vi "Format Commands to Tree.vi"(8 "Paths":path[](array[path])=[path "C:/Users/gam.AMER/Documents/2468 code/trunk/FRC/2019/Software/2019 robot/Drive/Commands/Drive for Time.vi", path "C:/Users/gam.AMER/Documents/2468 code/trunk/FRC/2019/Software/2019 robot/Drive/Commands/Drive Immediate.vi", path "C:/Users/gam.AMER/Documents/2468 code/trunk/FRC/2019/Software/2019 robot/Drive/Commands/J-Turn.vi", path "C:/Users/gam.AMER/Documents/2468 code/trunk/FRC/2019/Software/2019 robot/Drive/Commands/Play Path.vi", path "C:/Users/gam.AMER/Documents/2468 code/trunk/FRC/2019/Software/2019 robot/Drive/Commands/Read Drive Operation.vi", path "C:/Users/gam.AMER/Documents/2468 code/trunk/FRC/2019/Software/2019 robot/Drive/Commands/Reserve Drive.vi", path "C:/Users/gam.AMER/Documents/2468 code/trunk/FRC/2019/Software/2019 robot/Drive/Commands/Stop Driving.vi", path "C:/Users/gam.AMER/Documents/2468 code/trunk/FRC/2019/Software/2019 robot/Drive/Commands/Template for Drive Immediate with Deadband.vit", path "C:/Users/gam.AMER/Documents/2468 code/trunk/FRC/2019/Software/2019 robot/Drive/Commands/Template for Drive Immediate.vit", path "C:/Users/gam.AMER/Documents/2468 code/trunk/FRC/2019/Software/2019 robot/Drive/Commands/Template for Drive with Duration.vit", path "C:/Users/gam.AMER/Documents/2468 code/trunk/FRC/2019/Software/2019 robot/Climb/Commands/climb.vi", path "C:/Users/gam.AMER/Documents/2468 code/trunk/FRC/2019/Software/2019 robot/Climb/Commands/Read Climb Operation.vi", path "C:/Users/gam.AMER/Documents/2468 code/trunk/FRC/2019/Software/2019 robot/Climb/Commands/Reserve Climb.vi", path "C:/Users/gam.AMER/Documents/2468 code/trunk/FRC/2019/Software/2019 robot/Climb/Commands/Template for Climb Immediate with Deadband.vit", path "C:/Users/gam.AMER/Documents/2468 code/trunk/FRC/2019/Software/2019 robot/Climb/Commands/Template for Climb Immediate.vit", path "C:/Users/gam.AMER/Documents/2468 code/trunk/FRC/2019/Software/2019 robot/Climb/Commands/Template for Climb with Duration.vit", path "C:/Users/gam.AMER/Documents/2468 code/trunk/FRC/2019/Software/2019 robot/Elevator/Commands/Elevator Immediate.vi", path "C:/Users/gam.AMER/Documents/2468 code/trunk/FRC/2019/Software/2019 robot/Elevator/Commands/Read Elevator Operation.vi", path "C:/Users/gam.AMER/Documents/2468 code/trunk/FRC/2019/Software/2019 robot/Elevator/Commands/Reserve Elevator.vi", path "C:/Users/gam.AMER/Documents/2468 code/trunk/FRC/2019/Software/2019 robot/Elevator/Commands/Template for Elevator Immediate with Deadband.vit", path "C:/Users/gam.AMER/Documents/2468 code/trunk/FRC/2019/Software/2019 robot/Elevator/Commands/Template for Elevator Immediate.vit", path "C:/Users/gam.AMER/Documents/2468 code/trunk/FRC/2019/Software/2019 robot/Elevator/Commands/Template for Elevator with Duration.vit", path "C:/Users/gam.AMER/Documents/2468 code/trunk/FRC/2019/Software/2019 robot/Floating Intake/Commands/Duration Intake.vi", path "C:/Users/gam.AMER/Documents/2468 code/trunk/FRC/2019/Software/2019 robot/Floating Intake/Commands/Floating Intake Immediate.vi", path "C:/Users/gam.AMER/Documents/2468 code/trunk/FRC/2019/Software/2019 robot/Floating Intake/Commands/Floating Intake Read.vi", path "C:/Users/gam.AMER/Documents/2468 code/trunk/FRC/2019/Software/2019 robot/Floating Intake/Commands/Read Floating Intake Operation.vi", path "C:/Users/gam.AMER/Documents/2468 code/trunk/FRC/2019/Software/2019 robot/Floating Intake/Commands/Reserve Floating Intake.vi", path "C:/Users/gam.AMER/Documents/2468 code/trunk/FRC/2019/Software/2019 robot/Floating Intake/Commands/Template for Floating Intake Immediate with Deadband.vit", path "C:/Users/gam.AMER/Documents/2468 code/trunk/FRC/2019/Software/2019 robot/Floating Intake/Commands/Template for Floating Intake Immediate.vit", path "C:/Users/gam.AMER/Documents/2468 code/trunk/FRC/2019/Software/2019 robot/Floating Intake/Commands/Template for Floating Intake with Duration.vit", path "C:/Users/gam.AMER/Documents/2468 code/trunk/FRC/2019/Software/2019 robot/Carriage Intake/Commands/Carriage Intake Immediate with Deadband.vi", path "C:/Users/gam.AMER/Documents/2468 code/trunk/FRC/2019/Software/2019 robot/Carriage Intake/Commands/Carriage Intake Immediate.vi", path "C:/Users/gam.AMER/Documents/2468 code/trunk/FRC/2019/Software/2019 robot/Carriage Intake/Commands/Read Carriage Intake Operation.vi", path "C:/Users/gam.AMER/Documents/2468 code/trunk/FRC/2019/Software/2019 robot/Carriage Intake/Commands/Reserve Carriage Intake.vi", path "C:/Users/gam.AMER/Documents/2468 code/trunk/FRC/2019/Software/2019 robot/Carriage Intake/Commands/Template for Carriage Intake Immediate with Deadband.vit", path "C:/Users/gam.AMER/Documents/2468 code/trunk/FRC/2019/Software/2019 robot/Carriage Intake/Commands/Template for Carriage Intake Immediate.vit", path "C:/Users/gam.AMER/Documents/2468 code/trunk/FRC/2019/Software/2019 robot/Carriage Intake/Commands/Template for Carriage Intake with Duration.vit", path "C:/Users/gam.AMER/Documents/2468 code/trunk/FRC/2019/Software/2019 robot/LattePanda/Commands/Is Connected.vi", path "C:/Users/gam.AMER/Documents/2468 code/trunk/FRC/2019/Software/2019 robot/LattePanda/Commands/Power On.vi", path "C:/Users/gam.AMER/Documents/2468 code/trunk/FRC/2019/Software/2019 robot/LattePanda/Commands/Read LattePanda Operation.vi", path "C:/Users/gam.AMER/Documents/2468 code/trunk/FRC/2019/Software/2019 robot/LattePanda/Commands/Reserve LattePanda.vi", path "C:/Users/gam.AMER/Documents/2468 code/trunk/FRC/2019/Software/2019 robot/LattePanda/Commands/Shut Down.vi", path "C:/Users/gam.AMER/Documents/2468 code/trunk/FRC/2019/Software/2019 robot/LattePanda/Commands/Template for LattePanda Immediate with Deadband.vit", path "C:/Users/gam.AMER/Documents/2468 code/trunk/FRC/2019/Software/2019 robot/LattePanda/Commands/Template for LattePanda Immediate.vit", path "C:/Users/gam.AMER/Documents/2468 code/trunk/FRC/2019/Software/2019 robot/LattePanda/Commands/Template for LattePanda with Duration.vit"], 9 "Command Info":T4(array[cluster]), 11 "Tree Refnum":refnum<vi>) -> (2 "2D Picture":picture, 3 "Filtered Command Info Out":T1)   [LabVIEW 2019]
uses:
  <vilib>/picture/picture.llb/imagedata.ctl
  Command Editor Info.ctl
  Single Cmd Info.ctl
  <vilib>/Utility/Data Type/NI_Data Type.lvlib
panel:
  in  "Tree":string(tree)
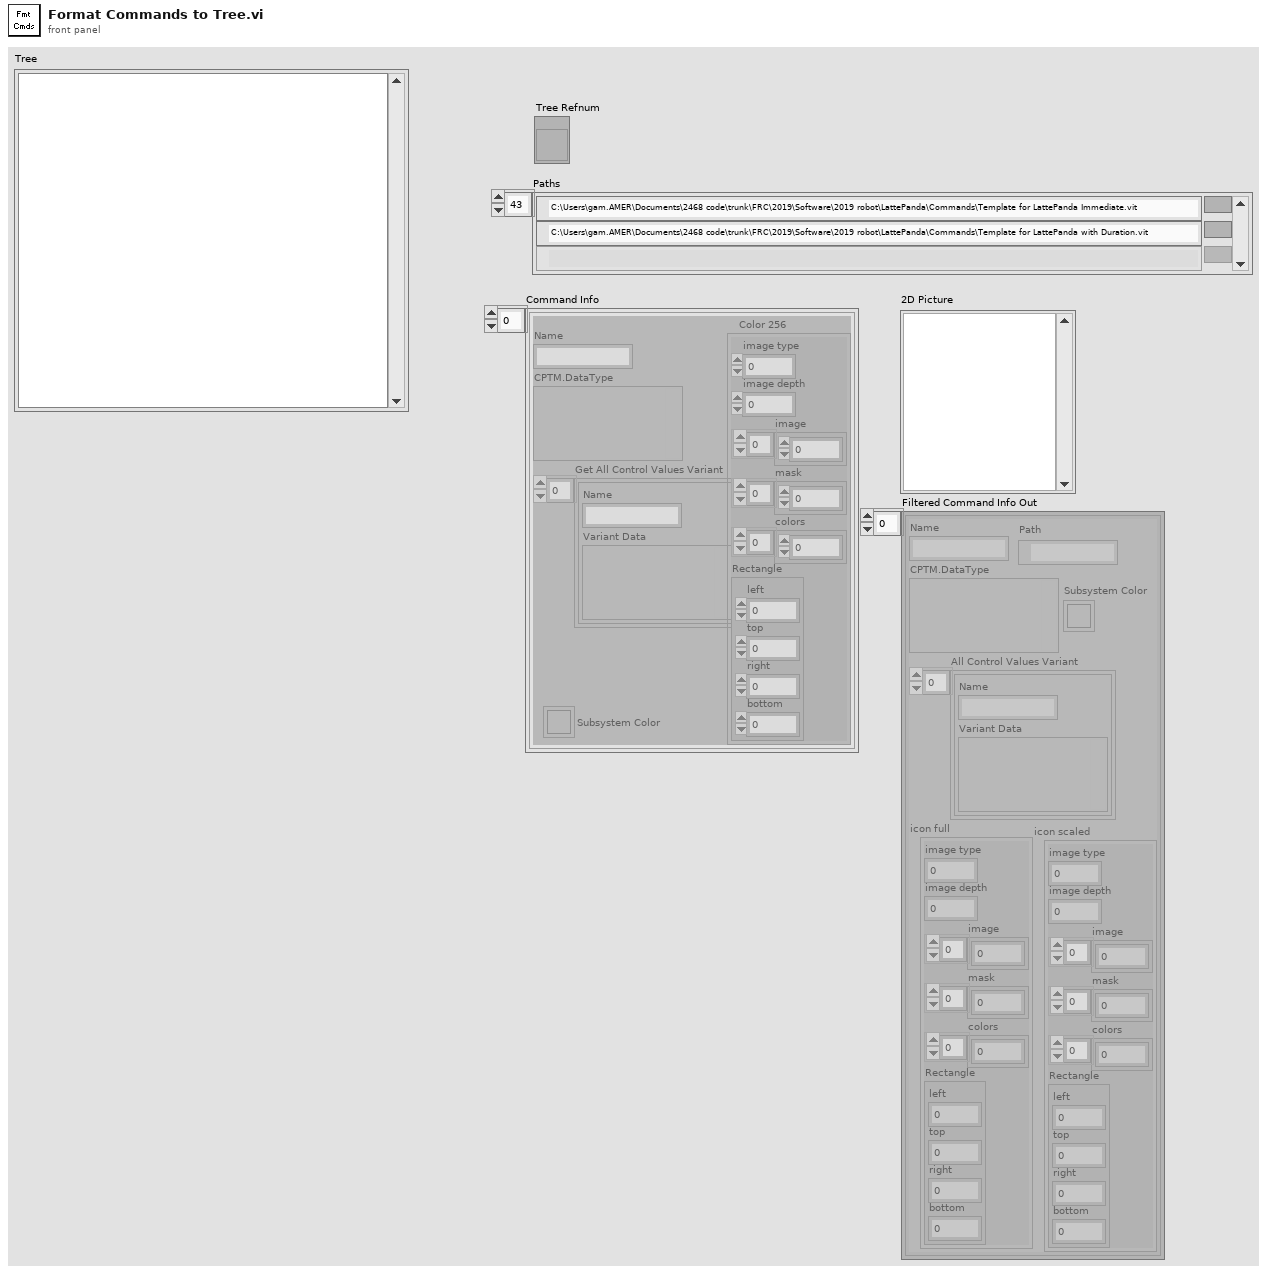
[diagram p1: front panel]
types:
  T1 = typedef "Command Editor Info.ctl" = T2[]
  T2 = typedef "Single Cmd Info.ctl" = cluster{"Name":string, "CPTM.DataType":variant, "All Control Values Variant":cluster{"Name":string, "Variant Data":variant}[], "icon full":T3, "icon scaled":T3, "Path":path, "Subsystem Color":u32}
  T3 = typedef "imagedata.ctl" = cluster{"image type":i32, "image depth":i32, "image":u8[], "mask":u8[], "colors":u32[], "Rectangle":cluster{"left":i16, "top":i16, "right":i16, "bottom":i16}}
  T4 = cluster{"Name":string, "CPTM.DataType":variant, "Get All Control Values Variant":cluster{"Name":string, "Variant Data":variant}[], "Color 256":T3, "Subsystem Color":u32}[]
  T5 = cluster{"Left Cell String":string, "Child Text":string[], "Child Tag":string, "Item Indent":i32, "Child Only?":bool, "Glyph Index":i32}
  T6 = cluster{"Left Cell String":string, "Child Text":string[], "Child Tag":string, "Item Indent":i32, "Child Only?":bool, "Glyph Index":i32}[]
  T7 = cluster{"Name":string, "CPTM.DataType":variant, "Get All Control Values Variant":cluster{"Name":string, "Variant Data":variant}[], "Color 256":T3, "Color 256":T3, "Local path":path, "Subsystem Color":u32}
  T8 = typedef "NI_Data Type.lvlib/Data Type.ctl" = enum8{"Invalid Type", "Void", "I8", "I16", "I32", "I64", "U8", "U16", "U32", "U64", "Single Float", "Double Float", "Extended Float", "Single Complex", "Double Complex", "Extended Complex", "Enum U8", "Enum U16", "Enum U32", "Enum U64", "Single Float With Unit", "Double Float With Unit", "Extended Float With Unit", "Single Complex with Unit", "Double Complex with Unit", "Extended Complex with Unit", "Boolean", "String", "Path", "Picture", "Tag", "Array", "Cluster", "Variant", "LV Variant", "Waveform", "Timestamp", "Digital Waveform", "Digital Data", "ExpressData", "Refnum", "External Data", "VI", "Poly VI", "LabVIEW Class Instance", "Fixed Point", "Set Collection", "Map Collection"}
  T9 = typedef "NI_Data Type.lvlib/Type Definition Info.ctl" = cluster{"Name":string, "Timestamp":u32}
  T10 = cluster{"left":i16, "top":i16, "right":i16, "bottom":i16}
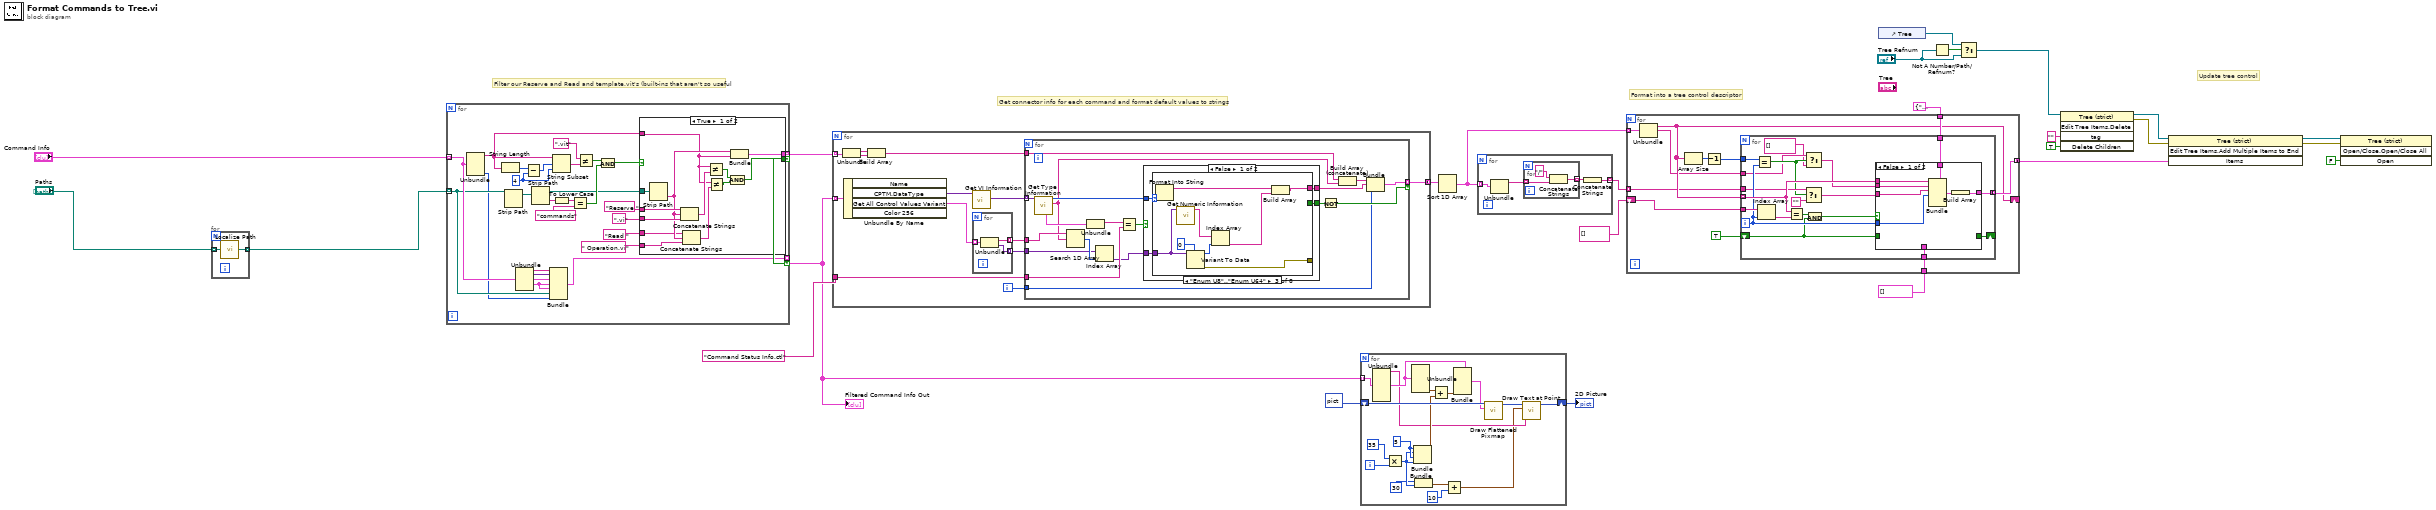
[diagram p0: block diagram]
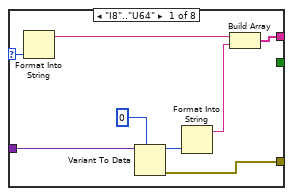
[diagram p3: hidden frame]
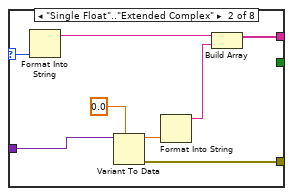
[diagram p4: hidden frame]
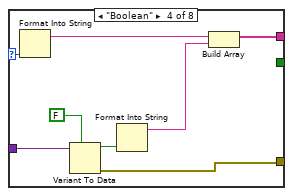
[diagram p5: hidden frame]
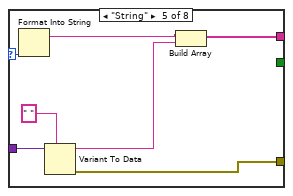
[diagram p6: hidden frame]
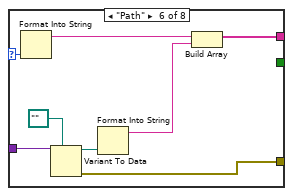
[diagram p7: hidden frame]
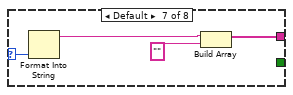
[diagram p8: hidden frame]
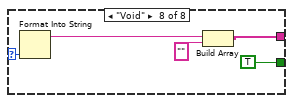
[diagram p9: hidden frame]
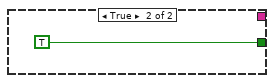
[diagram p10: hidden frame]
diagram:
  # "Update tree control"
  # "Get connector info for each command and format default values to strings"
  # "Filter our Reserve and Read and template.vit's (built-ins that aren't so useful"
  # "Format into a tree control descriptor"
  n1 = for {
    tunnel: "Paths" -> [w28] mode=indexing
    tunnel: [w27] -> w1 mode=indexing
    n2 = call "Localize Path.vi"("Path"=w28) -> ("Local path"=w27:path)
  }
  n3 = for {
    tunnel: "Command Info" -> [w31] mode=indexing
    tunnel: w1 -> [w30] mode=indexing
    tunnel: [w43] -> w4 mode=indexing if=w41
    tunnel: [w32] -> w3 mode=indexing if=w41
    w54 = 4
    n4 = Unbundle(w31) -> ("Name"=w42:string, "Subsystem Color"=w29:u32)  [unwired: 3 out]
    n5 = String Length(string=w42) -> (length=w56:i32)
    n6 = Strip Path(path=w30) -> (stripped path=w50:path)  [unwired: 1 out]
    n7 = Unbundle(w31) -> ("Name"=w33:string, "CPTM.DataType"=w34:variant, "Get All Control Values Variant"=w35:cluster{"Name":string, "Variant Data":variant}[], "Color 256"=w36:T3)  [unwired: 1 out]
    n8 = Subtract(x=w56, y=w54) -> (x-y=w55:i32)
    n9 = Strip Path(path=w50) -> (stripped path=w44:path, name=w49:string)
    n10 = Bundle("Name"=w33, "CPTM.DataType"=w34, "Get All Control Values Variant"=w35, "Color 256"=w36, "Color 256"=w36, "Local path"=w30, "Subsystem Color"=w29) -> (w32:T7)  [unwired: 1 in]
    n11 = String Subset(string=w42, offset (0)=w55, length (rest)=w54) -> (substring=w53:string)
    n12 = To Lower Case(string=w49) -> (all lower case string=w47:string)
    n13 = Equal?(x=w47, y="commands") -> (x = y?=w46:bool)
    n14 = Not Equal?(x=".vit", y=w53) -> (x != y?=w51:bool)
    n15 = Compound Arithmetic op=AND(w51, w46) -> (w45:bool)
    n16 = case shown="True" w45 {
      tunnel: w44 -> [w69 _]
      tunnel: w42 -> [w61 _]
      tunnel: [w68 _] -> w43
      tunnel: [w57 _] -> w41
      tunnel: "Reserve " -> [w67 _]
      tunnel: ".vi" -> [w66 _]
      tunnel: "Read " -> [w63 _]
      tunnel: " Operation.vi" -> [w62 _]
      frame True {
        n17 = Strip Path(path=w69) -> (name=w64:string)  [unwired: 1 out]
        n18 = Concatenate Strings(w67, w64, w66) -> (w65:string)
        n19 = Concatenate Strings(w63, w64, w62) -> (w60:string)
        n20 = Not Equal?(x=w61, y=w65) -> (x != y?=w58:bool)
        n21 = Not Equal?(x=w61, y=w60) -> (x != y?=w59:bool)
        n22 = Bundle("name"=w64, "Name"=w61) -> (w68:cluster{"name":string, "Name":string})  [unwired: 1 in]
        n23 = Compound Arithmetic op=AND(w58, w59) -> (w57:bool)
      }
      frame False {
      }
    }
  }
  "Filtered Command Info Out" <- w3
  n24 = for {
    tunnel: w4 -> [w82] mode=indexing
    tunnel: [w75] -> w23 mode=concatenating
    tunnel: w3 -> [w79] mode=indexing
    tunnel: "Command Status Info.ctl" ("Name") -> [w74]
    i -> [w70]
    n25 = Unbundle(w82) -> ("name"=w81:string, "Name"=w80:string)
    n26 = Unbundle By Name(w79) -> ("CPTM.DataType"=w78:variant, "Get All Control Values Variant"=w73:cluster{"Name":string, "Variant Data":variant}[])  [unwired: 2 out]
    n27 = Build Array(w81, w80) -> (w77:string[])
    n28 = call <vilib>:"Get VI Information.vi"("variant"=w78) -> ("VI terminal types"=w76:variant[])  [unwired: 7 in, 3 out]
    n29 = for {
      tunnel: w73 -> [w85] mode=indexing
      tunnel: [w84] -> w72 mode=indexing
      tunnel: [w83] -> w71 mode=indexing
      n30 = Unbundle(w85) -> ("Name"=w84:string, "Variant Data"=w83:variant)
    }
    n31 = for {
      tunnel: w77 -> [w101]
      tunnel: w76 -> [w103] mode=indexing
      tunnel: [w99] -> w75 mode=indexing if=w93
      tunnel: w74 -> [w97]
      tunnel: w72 -> [w91]
      tunnel: w71 -> [w88]
      tunnel: w70 -> [w86]
      n32 = call <vilib>:"Get Type Information.vi"("variant"=w103) -> ("name"=w90:string, "type"=w102:T8, "type definition info"=w98:T9)  [unwired: 6 in, 2 out]
      n33 = Search 1D Array(1D array=w91, element=w90) -> (index of element=w89:i32)  [unwired: 1 in]
      n34 = Unbundle(w98) -> ("Name"=w96:string)  [unwired: 1 out]
      n35 = Index Array(array=w88, index=w89) -> (element=w87:variant)
      n36 = Equal?(x=w96, y=w97) -> (x = y?=w95:bool)
      n37 = case shown="False" w95 {
        tunnel: w102 -> [w107 _]
        tunnel: [w106 _] -> w92
        tunnel: [w105 TRUE] -> w94
        tunnel: w87 -> [w104 _]
        frame False {
          n38 = case shown="\"Enum U8\"..\"Enum U64\"" w107 {
            selector: w107 -> [w115 w123 w132 w140 w147 w155 w159 w164]
            tunnel: [w110 w117 w129 w135 w144 w150 w157 w161] -> w106
            tunnel: [_ _ _ _ _ _ _ TRUE] -> w105
            tunnel: w104 -> [w109 w120 w127 w137 w146 w152 _ _]
            tunnel: [w108 w116 w128 w133 w141 w148 _ _] -> _
            frame "I8".."U64" {
              n39 = Format Into String(w115) -> (resulting string=w111:string)  [unwired: 3 in, 1 out]
              n40 = Variant To Data(type=i64 0, Variant=w109) -> (data=w113:i64, error out=w108:errorcluster)  [unwired: 1 in]
              n41 = Format Into String(w113) -> (resulting string=w112:string)  [unwired: 3 in, 1 out]
              n42 = Build Array(w111, w112) -> (w110:string[])
            }
            frame "Single Float".."Extended Complex" {
              n43 = Format Into String(w123) -> (resulting string=w119:string)  [unwired: 3 in, 1 out]
              n44 = Variant To Data(type=0.0, Variant=w120) -> (data=w121:dbl, error out=w116:errorcluster)  [unwired: 1 in]
              n45 = Format Into String(w121) -> (resulting string=w118:string)  [unwired: 3 in, 1 out]
              n46 = Build Array(w119, w118) -> (w117:string[])
            }
            frame "Enum U8".."Enum U64" {
              n47 = Format Into String(w132) -> (resulting string=w130:string)  [unwired: 3 in, 1 out]
              n48 = call <vilib>:"Get Numeric Information.vi"("variant"=w127) -> ("enum names"=w126:string[])  [unwired: 7 in, 3 out]
              n49 = Variant To Data(type=i64 0, Variant=w127) -> (data=w125:i64, error out=w128:errorcluster)  [unwired: 1 in]
              n50 = Index Array(array=w126, index=w125) -> (element=w124:string)
              n51 = Build Array(w130, w124) -> (w129:string[])
            }
            frame "Boolean" {
              n52 = Format Into String(w140) -> (resulting string=w136:string)  [unwired: 3 in, 1 out]
              n53 = Variant To Data(type=FALSE, Variant=w137) -> (data=w138:bool, error out=w133:errorcluster)  [unwired: 1 in]
              n54 = Format Into String(w138) -> (resulting string=w134:string)  [unwired: 3 in, 1 out]
              n55 = Build Array(w136, w134) -> (w135:string[])
            }
            frame "String" {
              n56 = Format Into String(w147) -> (resulting string=w145:string)  [unwired: 3 in, 1 out]
              n57 = Variant To Data(type=" ", Variant=w146) -> (data=w143:string, error out=w141:errorcluster)  [unwired: 1 in]
              n58 = Build Array(w145, w143) -> (w144:string[])
            }
            frame "Path" {
              n59 = Format Into String(w155) -> (resulting string=w151:string)  [unwired: 3 in, 1 out]
              n60 = Variant To Data(type=path "", Variant=w152) -> (data=w153:path, error out=w148:errorcluster)  [unwired: 1 in]
              n61 = Format Into String(w153) -> (resulting string=w149:string)  [unwired: 3 in, 1 out]
              n62 = Build Array(w151, w149) -> (w150:string[])
            }
            frame Default {
              n63 = Format Into String(w159) -> (resulting string=w158:string)  [unwired: 3 in, 1 out]
              n64 = Build Array(w158, "") -> (w157:string[])
            }
            frame "Void" {
              n65 = Format Into String(w164) -> (resulting string=w162:string)  [unwired: 3 in, 1 out]
              n66 = Build Array(w162, "") -> (w161:string[])
            }
          }
        }
        frame True {
        }
      }
      n67 = Not(x=w94) -> (.not. x?=w93:bool)
      n68 = Build Array (concatenate)(w101, w90) -> (w100:string[])
      n69 = Bundle(w100, w92, w86) -> (w99:cluster{string[], string[], i32})  [unwired: 1 in]
    }
  }
  n70 = for {
    tunnel: w3 -> [w182] mode=indexing
    shift-right: [w173] -> w5
    shift-left: picture data[5B] ("2D Picture") -> [w183]
    i -> [w178]
    w177 = 5
    n71 = Unbundle(w182) -> ("Name"=w169:string, "Color 256"=w181:T3)  [unwired: 5 out]
    n72 = Multiply(x=35, y=w178) -> (x*y=w171:i32)
    n73 = Unbundle(w181) -> ("Rectangle"=w179:T10)  [unwired: 5 out]
    n74 = Bundle(w177, w171, w177, w171) -> (w176:cluster{i32, i32, i32, i32})  [unwired: 1 in]
    n75 = Bundle(30, w171) -> (w168:cluster{i32, i32})  [unwired: 1 in]
    n76 = Add(x=w179, y=w176) -> (x+y=w175:cluster{i32, i32, i32, i32})
    n77 = Add(x=w168, y=10) -> (x+y=w167:cluster{i32, i32})
    n78 = Bundle(cluster=w181, "Rectangle"=w175) -> (w180:T3)  [unwired: 5 in]
    n79 = call <vilib>:"Draw Flattened Pixmap.vi"("image data"=w180, "picture"=w183) -> ("new picture"=w174:picture)  [unwired: 7 in]
    n80 = call <vilib>:"Draw Text at Point.vi"("text"=w169, "origin"=w167, "picture"=w174) -> ("new picture"=w173:picture)  [unwired: 7 in, 1 out]
  }
  "2D Picture" <- w5
  n81 = Sort 1D Array(array=w23) -> (sorted array=w24:cluster{string[], string[], i32}[])
  n82 = for {
    tunnel: w24 -> [w187] mode=indexing
    tunnel: [w184] -> w25 mode=indexing
    n83 = Unbundle(w187) -> (w186:string[])  [unwired: 2 out]
    n84 = for {
      tunnel: w186 -> [w189] mode=indexing
      tunnel: [w188] -> w185 mode=indexing
      n85 = Concatenate Strings("/", w189) -> (w188:string)
    }
    n86 = Concatenate Strings(w185) -> (w184:string)
  }
  n87 = for {
    tunnel: [w197] -> w26 mode=concatenating
    tunnel: T5 {"Left Cell String"="", "Child Text"=[], "Child Tag"="", "Item Indent"=0, "Child Only?"=FALSE, "Glyph Index"=0} ("Item") -> [w198]
    shift-right: [w194] -> _
    shift-left: string[] [] ("Child Text") -> [w200]
    tunnel: w24 -> [w201] mode=indexing
    tunnel: T6 [] -> [w199]
    tunnel: w25 -> [w193] mode=indexing
    n88 = Unbundle(w201) -> (w194:string[], w191:string[])  [unwired: 1 out]
    n89 = Array Size(array=w194) -> (size(s)=w196:i32)
    n90 = Decrement(x=w196) -> (x-1=w195:i32)
    n91 = for {
      tunnel: w200 -> [w220]
      tunnel: w194 -> [w215] mode=indexing
      tunnel: w199 -> [w218]
      tunnel: [w217] -> w197 mode=concatenating
      tunnel: w198 -> [w216]
      tunnel: w195 -> [w213]
      tunnel: w191 -> [w203]
      tunnel: w193 -> [w211]
      shift-right: [w207] -> _
      shift-left: TRUE -> [w206]
      i -> [w214]
      n92 = Equal?(x=w213, y=w214) -> (x = y?=w204:bool)
      n93 = Index Array(array=w220, index=w214) -> (element=w219:string)
      n94 = Equal?(x=w215, y=w219) -> (x = y?=w209:bool)
      n95 = Select(t=w211, s=w204, f="") -> (s? t:f=w212:string)
      n96 = Select(t=w203, s=w204, f=string[] [] ("appended array")) -> (s? t:f=w205:string[])
      n97 = And(x=w209, y=w206) -> (x .and. y?=w208:bool)
      n98 = case shown="False" w208 {
        tunnel: [w225 w229] -> w217
        tunnel: w218 -> [_ w229]
        tunnel: w216 -> [w227 _]
        tunnel: w215 -> [w224 _]
        tunnel: w214 -> [w223 _]
        tunnel: w205 -> [w222 _]
        tunnel: w212 -> [w221 _]
        tunnel: [_ w228] -> w207
        tunnel: w206 -> [_ w228]
        frame False {
          n99 = Bundle(cluster=w227, "Left Cell String"=w224, "Child Text"=w222, "Child Tag"=w221, "Item Indent"=w223) -> (w226:T5)  [unwired: 2 in]
          n100 = Build Array(w226) -> (w225:T6)
        }
        frame True {
        }
      }
    }
  }
  n101 = control-ref of="Tree"() -> (w8:refnum<vi>)
  n102 = Not A Number/Path/Refnum?(number/path/refnum="Tree Refnum") -> (NaN/Path/Refnum?=w12:bool)
  n103 = Select(t=w8, s=w12, f="Tree Refnum") -> (s? t:f=w11:refnum<vi>)
  n104 = invoke on="Invoke Node" class="Tree (strict)" method="Edit Tree Items.Delete"(reference=w11, "tag"="" ("Tag"), "Delete Children"=TRUE ("Delete Children?")) -> (reference out=w10:refnum<vi>, error out=w17:errorcluster)  [unwired: 2 in, 3 out]
  n105 = invoke on="Invoke Node" class="Tree (strict)" method="Edit Tree Items.Add Multiple Items to End"(reference=w10, error in=w17, "Items"=w26) -> (reference out=w9:refnum<vi>, error out=w14:errorcluster)  [unwired: 1 in, 2 out]
  n106 = invoke on="Invoke Node" class="Tree (strict)" method="Open/Close.Open/Close All"(reference=w9, error in=w14, "Open"=FALSE ("Open?")) -> ()  [unwired: 1 in, 4 out]
